vi "Simple UDP - Receiver.vi"() -> ()   [LabVIEW 2025]
doc: "The UDP protocol differs from TCP in that there is no error-checking with the packets of information that are sent, and thus no guarantee whatsoever that an intended recipient will actually receive a given piece of data.\n\nUDP does offer the ability to \"broadcast\" data across a network--simply specify an IP Address of all ones (255.255.255.255) to attempt to broadcast information network-wide. Keep in mind that routers and other network hardware will generally refuse to forward the broadcast beyond certain points, so the extent of the broadcast will in practice be limited."
uses:
  StoprVar.vi
panel:
  out "CH3":dbl(graph) caption="CH 2"
  out "CH 5":dbl caption="Numeric" format="%#_6f"
  out "CH  4":dbl caption="Numeric" format="%#_6f"
  out "CH1":dbl caption="Numeric" format="%#_4f"
  out "CH 2":dbl caption="Numeric" format="%#_6f"
  out "CH3":dbl caption="Numeric" format="%#_6f"
  out "CH 6":dbl caption="Numeric" format="%#_6f"
  in  "Tab Control":enum32{"Main", "Config", "Debug"}(tab)
  in  "Stop 2":bool
  out "IP address":string
  in  "Run":bool
  in  "Stop":bool
  out "Status":bool=TRUE
  in  "STOP":bool
  in  "START":bool
  in  "Param 2":dbl format="%#_13g"
  in  "Param 3":dbl format="%#_13g"
  in  "Param 4":dbl format="%#_13g"
  in  "Param 5":dbl format="%#_13g"
  in  "Param 6":dbl format="%#_13g"
  in  "String 5":string="CH 6"
  in  "String 4":string="CH 5"
  in  "String 3":string="CH 4"
  in  "String 2":string="CH 2"
  in  "String":string="CH 3"
  in  "String":string="CH 1 "
  in  "Max":dbl=10.0
  in  "Min":dbl
  in  "Max":dbl=10.0
  in  "Min":dbl
  in  "Max":dbl=10.0
  in  "Min":dbl
  in  "Max":dbl=10.0
  in  "Min":dbl
  in  "Max":dbl=10.0
  in  "Min":dbl
  in  "Max":dbl=10.0
  in  "Min":dbl
  in  "address":string="192.168.1.12"
  in  "remote port":u16=25000
  in  "local port":u16=1888
  in  "receiver port":u16=54400
  in  "Apply":bool
  in  "Clear Chart":bool
  out "Recived Data (ASCII)":string
  out "CH 6":dbl(graph)
  out "CH 5":dbl(graph)
  out "CH 4":dbl(graph)
  out "CH2":dbl(graph) caption="CH 2"
  out "CH1":dbl(graph) caption="CH 1"
  # "Start | Stop |  EXIT GUI"
  # "Params"
  # "Converter"
  # "Network"
  # "Charts"
  # "Scaling"
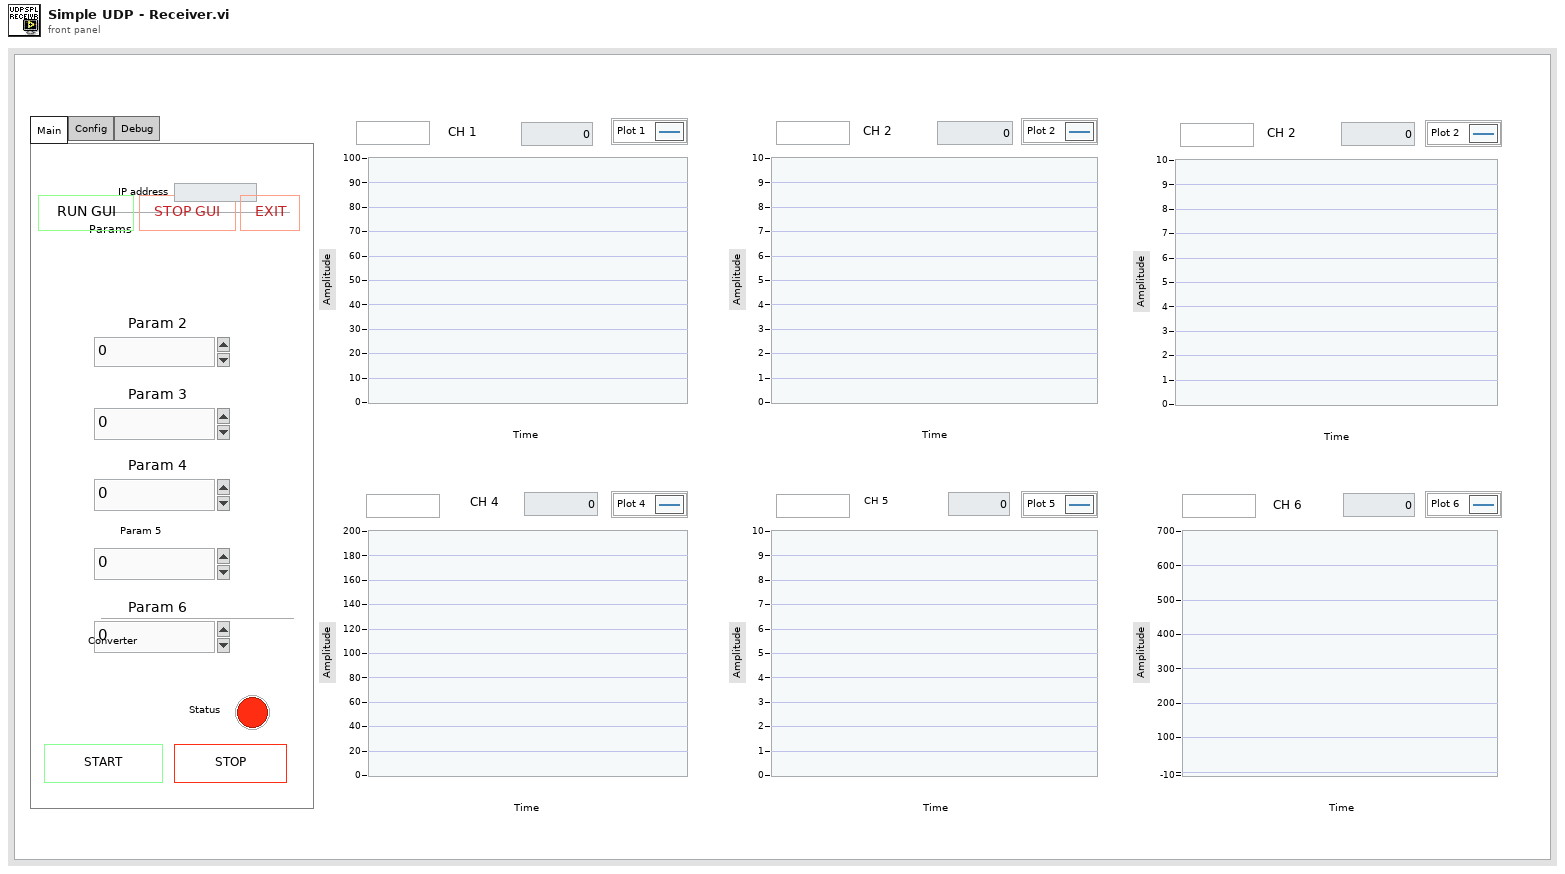
[diagram p1: front panel]
types:
  T1 = enum16{"big-endian, network order", "native, host order", "little-endian"}
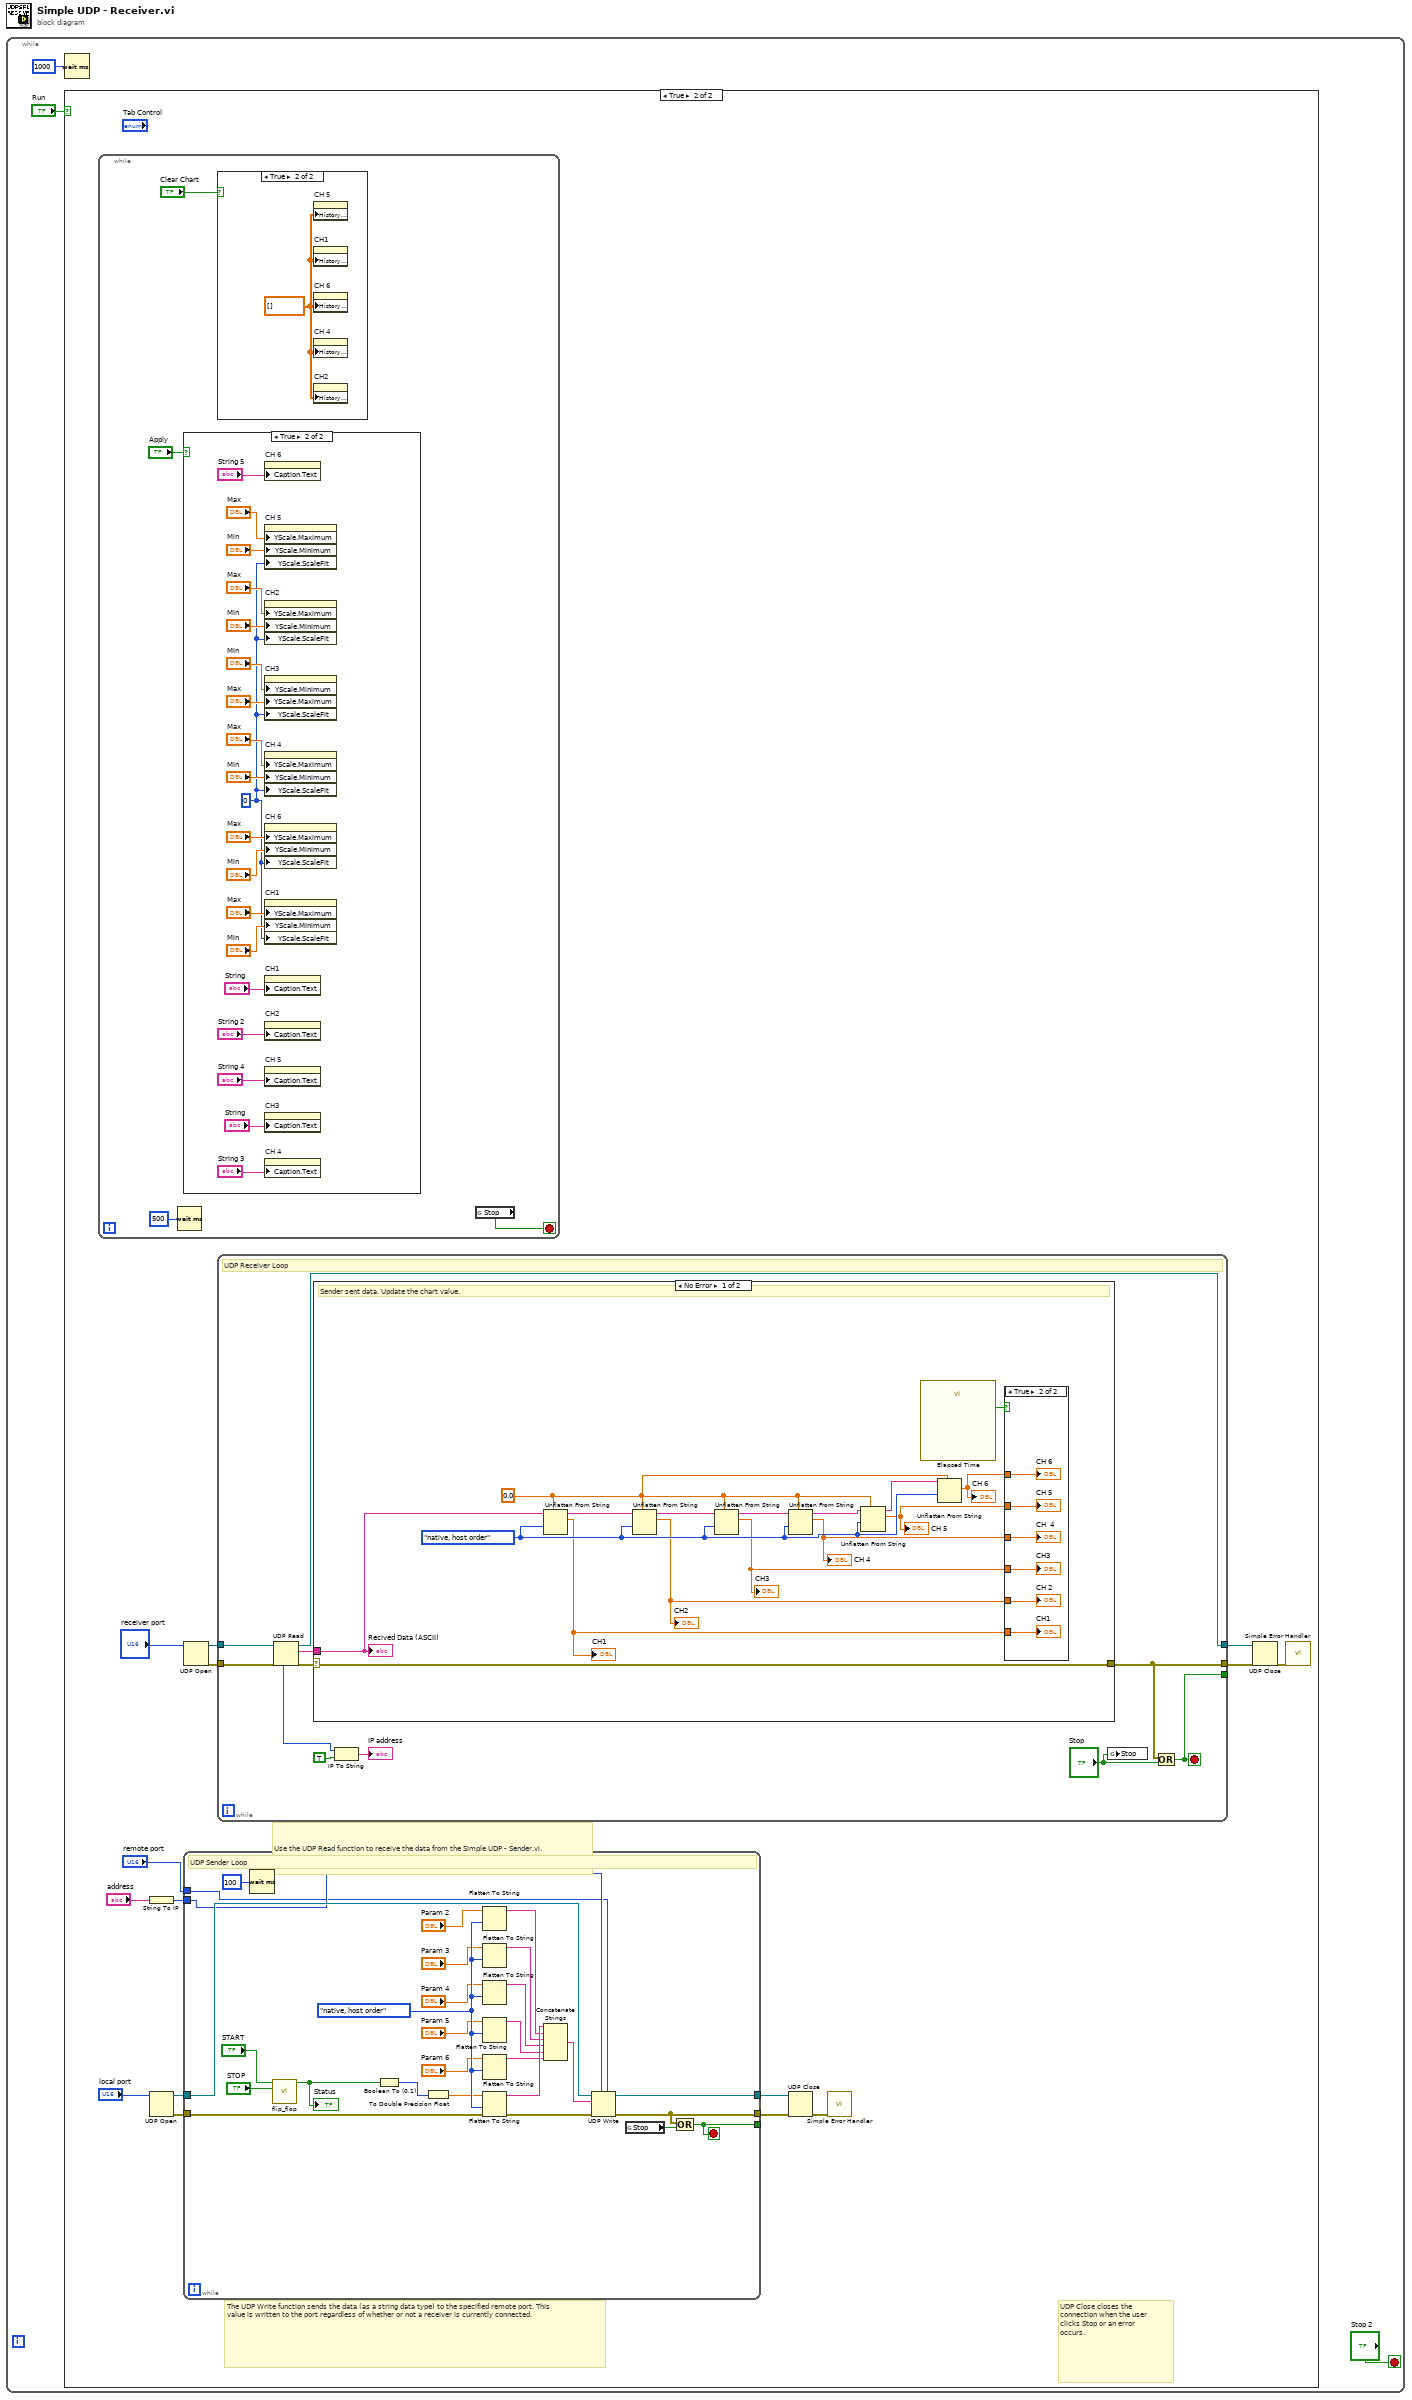
[diagram p0: block diagram]
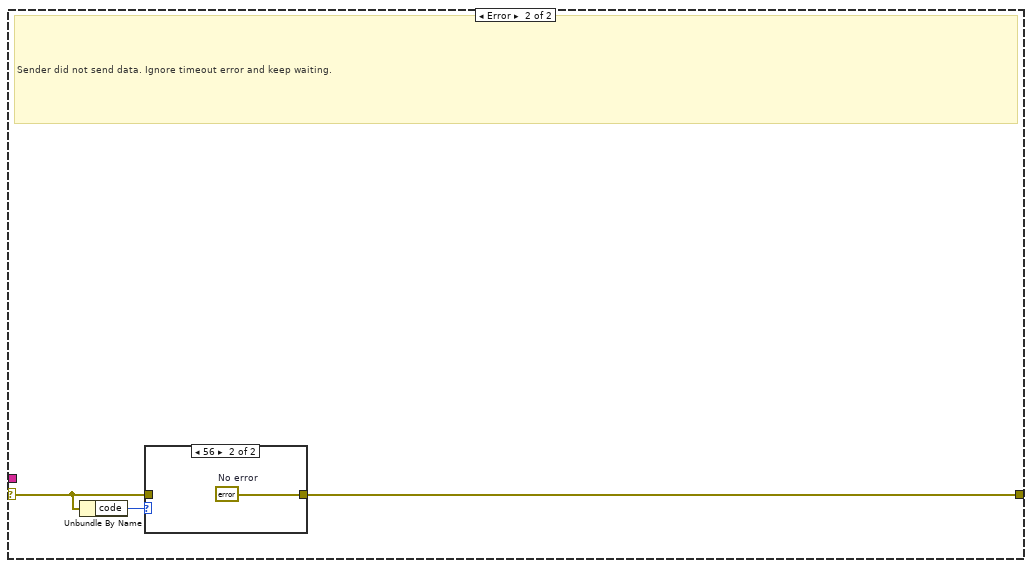
[diagram p6: hidden frame]
diagram:
  n1 = while {
    stop <- "Stop 2" stop-if-true
    n2 = Wait (ms)(milliseconds to wait=u32 1000) -> ()  [unwired: 1 out]
    n3 = case shown="True" "Run" {
      frame False {
      }
      frame True {
        # "The UDP Write function sends the data (as a string data type) to the specified remote port. This value is written to the port regardless of whether or not a receiver is currently connected."
        # "Use the UDP Read function to receive the data from the Simple UDP - Sender.vi."
        # "UDP Close closes the connection when the user clicks Stop or an error occurs."
        n4 = while {
          stop <- w22 stop-if-true
          n5 = Wait (ms)(milliseconds to wait=u32 500) -> ()  [unwired: 1 out]
          n6 = case shown="True" "Apply" {
            frame False {
            }
            frame True {
              w24 = u8 0 ("Y Scale.Scale Fit")
              n7 = property on="CH 6" class="WFChart (strict)"("Caption.Text"="String 5") -> ()  [unwired: 2 in, 2 out]
              n8 = property on="CH 5" class="WFChart (strict)"("YScale.Maximum"="Max", "YScale.Minimum"="Min", "YScale.ScaleFit"=w24) -> ()  [unwired: 2 in, 2 out]
              n9 = property on="CH2" class="WFChart (strict)"("YScale.Maximum"="Max", "YScale.Minimum"="Min", "YScale.ScaleFit"=w24) -> ()  [unwired: 2 in, 2 out]
              n10 = property on="CH3" class="WFChart (strict)"("YScale.Minimum"="Min", "YScale.Maximum"="Max", "YScale.ScaleFit"=w24) -> ()  [unwired: 2 in, 2 out]
              n11 = property on="CH 4" class="WFChart (strict)"("YScale.Maximum"="Max", "YScale.Minimum"="Min", "YScale.ScaleFit"=w24) -> ()  [unwired: 2 in, 2 out]
              n12 = property on="CH 6" class="WFChart (strict)"("YScale.Maximum"="Max", "YScale.Minimum"="Min", "YScale.ScaleFit"=w24) -> ()  [unwired: 2 in, 2 out]
              n13 = property on="CH1" class="WFChart (strict)"("YScale.Maximum"="Max", "YScale.Minimum"="Min", "YScale.ScaleFit"=w24) -> ()  [unwired: 2 in, 2 out]
              n14 = property on="CH1" class="WFChart (strict)"("Caption.Text"="String") -> ()  [unwired: 2 in, 2 out]
              n15 = property on="CH2" class="WFChart (strict)"("Caption.Text"="String 2") -> ()  [unwired: 2 in, 2 out]
              n16 = property on="CH 5" class="WFChart (strict)"("Caption.Text"="String 4") -> ()  [unwired: 2 in, 2 out]
              n17 = property on="CH3" class="WFChart (strict)"("Caption.Text"="String") -> ()  [unwired: 2 in, 2 out]
              n18 = property on="CH 4" class="WFChart (strict)"("Caption.Text"="String 3") -> ()  [unwired: 2 in, 2 out]
            }
          }
          n19 = case shown="True" "Clear Chart" {
            frame False {
            }
            frame True {
              w23 = dbl[] [] ("History Data")
              n20 = property on="CH 5" class="WFChart (strict)"("History Data"=w23) -> ()  [unwired: 2 in, 2 out]
              n21 = property on="CH1" class="WFChart (strict)"("History Data"=w23) -> ()  [unwired: 2 in, 2 out]
              n22 = property on="CH 6" class="WFChart (strict)"("History Data"=w23) -> ()  [unwired: 2 in, 2 out]
              n23 = property on="CH 4" class="WFChart (strict)"("History Data"=w23) -> ()  [unwired: 2 in, 2 out]
              n24 = property on="CH2" class="WFChart (strict)"("History Data"=w23) -> ()  [unwired: 2 in, 2 out]
            }
          }
          n25 = global read "StoprVar.vi" "Stop"() -> (w22:bool)
        }
        n26 = String To IP(1:"address") -> (0:w10:u32)
        n27 = UDP Open(11:"local port") -> (port=w11:refnum<k16>, 0:w12:errorcluster)  [unwired: 4 in, 1 out]
        n28 = UDP Open(11:"receiver port") -> (port=w14:refnum<k16>, 0:w15:errorcluster)  [unwired: 4 in, 1 out]
        n29 = while {
          tunnel: [w68] -> w8
          tunnel: w11 -> [w70]
          tunnel: w12 -> [w63]
          tunnel: [w69] -> w7
          tunnel: w10 -> [w67]
          tunnel: "remote port" -> [w65]
          tunnel: [w49] -> _
          stop <- w49 stop-if-true
          w54 = T1."native, host order" ("byte order (0:big-endian, network order)")
          # "UDP Sender Loop"
          n30 = Wait (ms)(milliseconds to wait=u32 100) -> ()  [unwired: 1 out]
          n31 = call "flip_flop.vi"("STOP"="STOP", "START"="START") -> ("Boolean"=w43:bool)  [unwired: 9 in]
          "Status" <- w43
          n32 = Boolean To (0,1)(Boolean=w43) -> (0, 1=w46:i16)
          n33 = To Double Precision Float(number=w46) -> (double precision float=w47:dbl)
          n34 = Flatten To String(anything="Param 2", byte order (0:big-endian, network order)=w54) -> (data string=w60:string)  [unwired: 2 in, 2 out]
          n35 = Flatten To String(anything="Param 3", byte order (0:big-endian, network order)=w54) -> (data string=w59:string)  [unwired: 2 in, 2 out]
          n36 = Flatten To String(anything="Param 4", byte order (0:big-endian, network order)=w54) -> (data string=w58:string)  [unwired: 2 in, 2 out]
          n37 = Flatten To String(anything="Param 5", byte order (0:big-endian, network order)=w54) -> (data string=w57:string)  [unwired: 2 in, 2 out]
          n38 = Flatten To String(anything="Param 6", byte order (0:big-endian, network order)=w54) -> (data string=w56:string)  [unwired: 2 in, 2 out]
          n39 = Flatten To String(anything=w47, byte order (0:big-endian, network order)=w54, error in (no error)=w63) -> (data string=w61:string, error out=w62:errorcluster)  [unwired: 1 in, 1 out]
          n40 = Concatenate Strings(w61, w60, w59, w58, w57, w56) -> (w64:string)
          n41 = UDP Write(address=w67, port or service name=w65, connection ID=w70, data in=w64, 8:w62) -> (error out=w68:errorcluster, 3:w69:refnum<k16>)  [unwired: 1 in]
          n42 = global read "StoprVar.vi" "Stop"() -> (w48:bool)
          n43 = Or(x=w68, y=w48) -> (x .or. y?=w49:bool)
        }
        n44 = while {
          tunnel: w14 -> [w81]
          tunnel: [w76] -> w18
          tunnel: w15 -> [w80]
          tunnel: [w77] -> w16
          tunnel: [w73] -> _
          stop <- w73 stop-if-true
          # "UDP Receiver Loop"
          n45 = UDP Read(connection ID=w81, 8:w80) -> (data out=w79:string, error out=w78:errorcluster, 3:w76:refnum<k16>, 6:w75:u32)  [unwired: 1 in, 2 out]
          n46 = case shown="No Error" w78 {
            selector: w78 -> [w97 w105]
            tunnel: w79 -> [w96 _]
            tunnel: [w97 w104] -> w77
            frame No Error {
              w89 = 0.0
              w90 = T1."native, host order" ("byte order (0:big-endian, network order)")
              # "Sender sent data. Update the chart value."
              n47 = Unflatten From String(type=w89, binary string=w96, byte order (0:big-endian, network order)=w90) -> (rest of the binary string=w95:string, value=w84:dbl)  [unwired: 2 in, 1 out]
              "CH1" <- w84
              n48 = Unflatten From String(type=w89, binary string=w95, byte order (0:big-endian, network order)=w90) -> (rest of the binary string=w94:string, value=w87:dbl)  [unwired: 2 in, 1 out]
              "CH2" <- w87
              n49 = Unflatten From String(type=w89, binary string=w94, byte order (0:big-endian, network order)=w90) -> (rest of the binary string=w93:string, value=w82:dbl)  [unwired: 2 in, 1 out]
              "CH3" <- w82
              n50 = Unflatten From String(type=w89, binary string=w93, byte order (0:big-endian, network order)=w90) -> (rest of the binary string=w92:string, value=w85:dbl)  [unwired: 2 in, 1 out]
              "CH 4" <- w85
              n51 = Unflatten From String(type=w89, binary string=w92, byte order (0:big-endian, network order)=w90) -> (rest of the binary string=w91:string, value=w88:dbl)  [unwired: 2 in, 1 out]
              "CH 5" <- w88
              n52 = call "Elapsed Time"() -> ("Time has Elapsed"=w83:bool)  [unwired: 12 in, 7 out]
              n53 = Unflatten From String(type=w89, binary string=w91, byte order (0:big-endian, network order)=w90) -> (value=w86:dbl)  [unwired: 2 in, 2 out]
              "CH 6" <- w86
              n54 = case shown="True" w83 {
                tunnel: w88 -> [_ w103]
                tunnel: w87 -> [_ w102]
                tunnel: w82 -> [_ w101]
                tunnel: w86 -> [_ w100]
                tunnel: w85 -> [_ w99]
                tunnel: w84 -> [_ w98]
                frame False {
                }
                frame True {
                  "CH 2" <- w102
                  "CH1" <- w98
                  "CH 6" <- w100
                  "CH3" <- w101
                  "CH  4" <- w99
                  "CH 5" <- w103
                }
              }
              "Recived Data (ASCII)" <- w96
            }
            frame Error {
              # "Sender did not send data. Ignore timeout error and keep waiting."
              n55 = Unbundle By Name(w105) -> ("code"=w106:i32)
              n56 = case shown="56" w106 {
                tunnel: w105 -> [w107 _]
                tunnel: [w107 w108] -> w104
                frame Default {
                }
                frame 56 {
                  w108 = errorcluster {"status"=FALSE, "code"=0, "source"=""}  # No error
                }
              }
            }
          }
          n57 = IP To String(1:TRUE ("dot notation? (F)"), 2:w75) -> (0:→"IP address":string)
          n58 = global write "StoprVar.vi" "Stop"("Stop") -> ()
          n59 = Or(x=w77, y="Stop") -> (x .or. y?=w73:bool)
        }
        n60 = UDP Close(connection ID=w7, 8:w8) -> (error out=w9:errorcluster)  [unwired: 1 out]
        n61 = call <vilib>:"Simple Error Handler.vi"("error in (no error)"=w9) -> ()  [unwired: 4 in, 5 out]
        n62 = UDP Close(connection ID=w18, 8:w16) -> (error out=w17:errorcluster)  [unwired: 1 out]
        n63 = call <vilib>:"Simple Error Handler.vi"("error in (no error)"=w17) -> ()  [unwired: 1 in, 8 out]
      }
    }
  }
